vi "Add Value Control to Cluster and Rename.vi"(8 "error in (no error)":errorcluster, 9 "New Label.Text":string, 10 "Private Data Refs":T1, 11 "GObject in":refnum<vi>) -> (0 "error out":errorcluster, 3 "GObject out":refnum<vi>)   [LabVIEW 2020, in "Add to Private Data.lvlib"]
uses:
  Add to Private Data.lvlib
  Private Data Refs.ctl
  <vilib>/Utility/miscctls.llb/LVPositionTypeDef.ctl
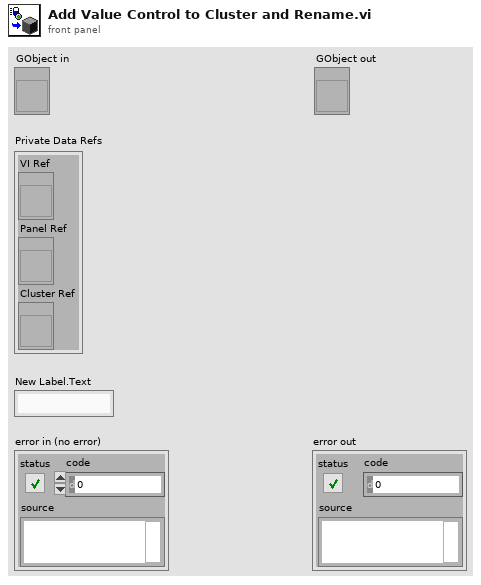
[diagram p1: front panel]
types:
  T1 = typedef "Add to Private Data.lvlib/Private Data Refs.ctl" = cluster{"VI Ref":refnum<vi>, "Panel Ref":refnum<vi>, "Cluster Ref":refnum<vi>}
  T2 = typedef "LVPositionTypeDef.ctl" = cluster{"Left":i32, "Top":i32}
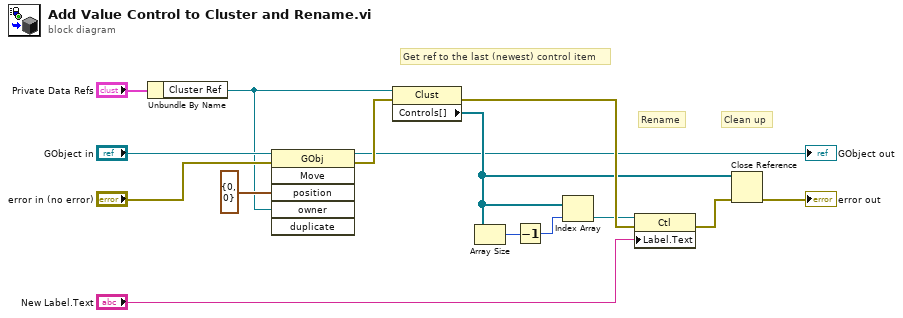
[diagram p0: block diagram]
diagram:
  # "Clean up"
  # "Rename"
  # "Get ref to the last (newest) control item"
  n1 = Unbundle By Name("Private Data Refs") -> ("Cluster Ref"=w2:refnum<vi>)
  n2 = invoke class="GObj" method="Move"(reference="GObject in", error in="error in (no error)", "position"=T2 {"Left"=0, "Top"=0}, "owner"=w2) -> (reference out=→"GObject out":refnum<vi>, error out=w13:errorcluster)  [unwired: 2 in, 4 out]
  n3 = property class="Clust"(reference=w2, error in=w13) -> (error out=w14:errorcluster, "Controls[]"=w8:refnum<vi>[])  [unwired: 1 out]
  n4 = Array Size(array=w8) -> (size(s)=w6:i32)
  n5 = Decrement(x=w6) -> (x-1=w7:i32)
  n6 = Index Array(array=w8, index=w7) -> (element=w9:refnum<vi>)
  n7 = property class="Ctl"(reference=w9, error in=w14, "Label.Text"="New Label.Text") -> (error out=w10:errorcluster)  [unwired: 1 out]
  n8 = Close Reference(reference=w8, error in (no error)=w10) -> (error out=→"error out":errorcluster)
